vi "abort-acquisition.vi"(3 "error in (no error)":errorcluster, 4 "Manufacturer":enum16{"Andor", "Xenics"}(ring), 5 "Cam Ref":T1) -> (0 "error out":errorcluster, 1 "aborted":bool, 2 "Cam Ref Out":T1)   [LabVIEW 2015]
uses:
  <vilib>/Xenics Infrared Solutions/Xeneth LabVIEW API/VIs/Controls/Camara.ctl
  <userlib>/atmcd32d.llb/Error Code Enum typedef.ctl
  <vilib>/Xenics Infrared Solutions/Xeneth LabVIEW API/Xeneth.lvlib
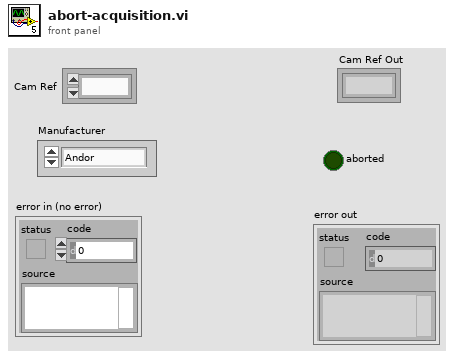
[diagram p1: front panel]
types:
  T1 = typedef "Xeneth.lvlib/Camara.ctl" = refnum<k1>
  T2 = typedef "Error Code Enum typedef.ctl" = enum32{"N/A (0)", "DRV_ERROR_CODES", "DRV_SUCCESS", "DRV_VXDNOTINSTALLED", "DRV_ERROR_SCAN", "DRV_ERROR_CHECK_SUM", "DRV_ERROR_FILELOAD", "DRV_UNKNOWN_FUNC", "DRV_ERROR_VXD_INIT", "DRV_ERROR_ADDRESS", "DRV_ERROR_PAGELOCK", "DRV_ERROR_PAGEUNLOCK", "DRV_ERROR_BOARDTEST", "DRV_ERROR_ACK", "DRV_ERROR_UP_FIFO", "DRV_ERROR_PATTERN", "N/A (16)", "DRV_ACQUISITION_ERRORS", "DRV_ACQ_BUFFER", "DRV_ACQ_DOWNFIFO_FULL", "DRV_PROC_UNKONWN_INSTRUCTION", "DRV_ILLEGAL_OP_CODE", "DRV_KINETIC_TIME_NOT_MET", "DRV_ACCUM_TIME_NOT_MET", "DRV_NO_NEW_DATA", "N/A (25)", "DRV_SPOOLERROR", "N/A (27)", "N/A (28)", "N/A (29)", "N/A (30)", "N/A (31)", "N/A (32)", "DRV_TEMPERATURE_CODES", "DRV_TEMPERATURE_OFF", "DRV_TEMPERATURE_NOT_STABILIZED", "DRV_TEMPERATURE_STABILIZED", "DRV_TEMPERATURE_NOT_REACHED", "DRV_TEMPERATURE_OUT_RANGE", "DRV_TEMPERATURE_NOT_SUPPORTED", "DRV_TEMPERATURE_DRIFT", "N/A (41)", "N/A (42)", "N/A (43)", "N/A (44)", "N/A (45)", "N/A (46)", "N/A (47)", "N/A (48)", "DRV_GENERAL_ERRORS", "DRV_INVALID_AUX", "DRV_COF_NOTLOADED", "DRV_FPGAPROG", "DRV_FLEXERROR", "DRV_GPIBERROR", "N/A (55)", "N/A (56)", "N/A (57)", "N/A (58)", "N/A (59)", "N/A (60)", "N/A (61)", "N/A (62)", "N/A (63)", "DRV_DATATYPE", "DRV_DRIVER_ERRORS", "DRV_P1INVALID", "DRV_P2INVALID", "DRV_P3INVALID", "DRV_P4INVALID", "DRV_INIERROR", "DRV_COFERROR", "DRV_ACQUIRING", "DRV_IDLE", "DRV_TEMPCYCLE", "DRV_NOT_INITIALIZED", "DRV_P5INVALID", "DRV_P6INVALID", "DRV_INVALID_MODE", "DRV_INVALID_FILTER", "DRV_I2CERRORS", "DRV_I2CDEVNOTFOUND", "DRV_I2CTIMEOUT", "DRV_P7INVALID", "N/A (84)", "N/A (85)", "N/A (86)", "N/A (87)", "N/A (88)", "N/A (89)", "DRV_IOCERROR", "DRV_VRMVERSIONERROR"}
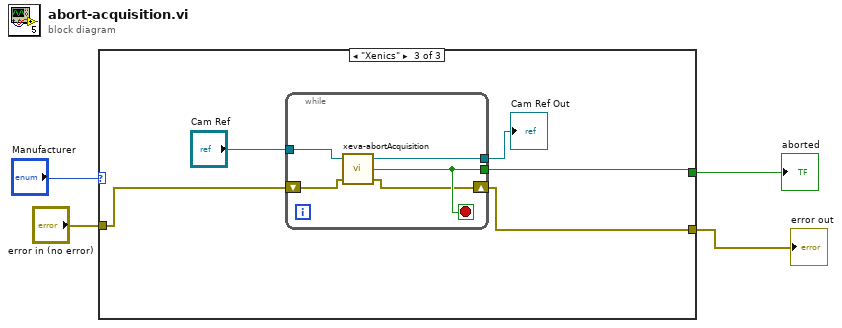
[diagram p0: block diagram]
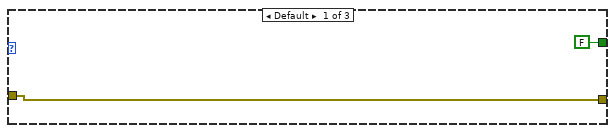
[diagram p2: hidden frame]
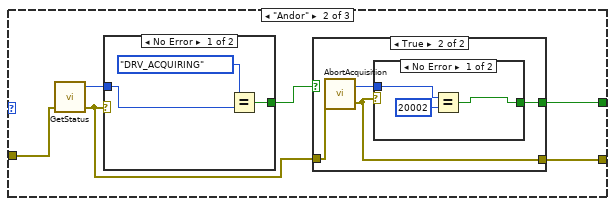
[diagram p3: hidden frame]
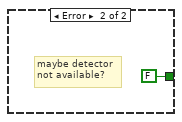
[diagram p4: hidden frame]
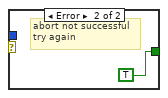
[diagram p6: hidden frame]
diagram:
  n1 = case shown="\"Xenics\"" "Manufacturer" {
    tunnel: [FALSE w10 w30] -> w4
    tunnel: "error in (no error)" -> [w5 w9 w29]
    tunnel: [w5 w7 w28] -> w1
    frame Default {
    }
    frame "Andor" {
      n2 = call <userlib>:"GetStatus.vi"("error in (no error)"=w9) -> ("error out"=w8:errorcluster, "status"=w11:T2)  [unwired: 2 in, 1 out]
      n3 = case shown="No Error" w8 {
        tunnel: w11 -> [w14 _]
        tunnel: [w13 FALSE] -> w12
        frame No Error {
          n4 = Equal?(x=Error_Code_Enum_typedef."DRV_ACQUIRING" ("Acquisition Status"), y=w14) -> (x = y?=w13:bool)
        }
        frame Error {
          # "maybe detector\nnot available?"
        }
      }
      n5 = case shown="True" w12 {
        selector: w12 -> [w18 _]
        tunnel: [w18 w21] -> w10
        tunnel: w8 -> [w17 w20]
        tunnel: [w17 w19] -> w7
        frame False {
        }
        frame True {
          n6 = call <userlib>:"AbortAcquisition.vi"("error in (no error)"=w20) -> ("error out"=w19:errorcluster, "DLL error code"=w22:u32)  [unwired: 1 in]
          n7 = case shown="No Error" w19 {
            tunnel: w22 -> [w24 _]
            tunnel: [w23 TRUE] -> w21
            frame No Error {
              n8 = Equal?(x=w24, y=u32 20002 ("= temperature\naccepted")) -> (x = y?=w23:bool)
            }
            frame Error {
              # "abort not successful\ntry again"
            }
          }
        }
      }
    }
    frame "Xenics" {
      n9 = while {
        tunnel: "Cam Ref" -> [w36]
        tunnel: [w35] -> w30
        shift-right: [w34] -> w28
        shift-left: w29 -> [w33]
        tunnel: [w32] -> w27
        stop <- w35 stop-if-true
        n10 = call "xeva-abortAcquisition.vi"("error in (no error)"=w33, "Cam Ref"=w36) -> ("error out"=w34:errorcluster, "aborted"=w35:bool, "Cam Ref Out"=w32:T1)  [unwired: 1 in]
      }
      "Cam Ref Out" <- w27
    }
  }
  "aborted" <- w4
  "error out" <- w1
